vi "ConfigTriggerRequest.vi"(8 "error in (no error)":errorcluster, 10 "TriggerParams":T1={"eTrigger"=0, "eEdge"=10280, "sSource"=""} {"eEdge" items=["Rising"=10280, "Falling"=10171]; "eTrigger" items=["None", "Digital", "Analog"]}, 11 "ModuleID":i32) -> (0 "error out":errorcluster)   [LabVIEW 2014, in "FGenPlugins.lvlib" / "NISTFGenPluginsBase.lvclass"]
uses:
  NISTFGenPluginsBase.lvclass
  TypeDef/TriggerParams.ctl
  FGenModule/Protected/clEventType.ctl
  <vilib>/Utility/error.llb/Error Cluster From Error Code.vi
  <vilib>/ErrorRing/Error Ring.xnode
  FGenModule/FGenModule.lvlib
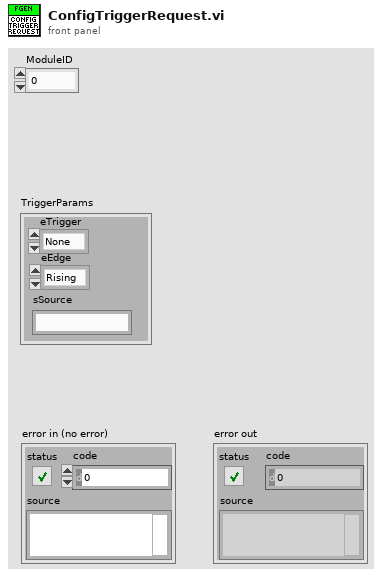
[diagram p1: front panel]
types:
  T1 = typedef "FGenPlugins.lvlib/NISTFGenPluginsBase.lvclass/TriggerParams.ctl" = cluster{"eTrigger":u16, "eEdge":u16, "sSource":string}
  T2 = typedef "FGenModule.lvlib/clRequestEvents.ctl" = cluster{"StopRequest":refnum<user-event>, "PathToINI":refnum<user-event>, " LoadPlugin":refnum<user-event>, "OperateMode":refnum<user-event>, "OutputEnable":refnum<user-event>, "OutputMode":refnum<user-event>, "RefClkSource":refnum<user-event>, "ChannelName":refnum<user-event>, "Generation":refnum<user-event>, "AbortGeneration":refnum<user-event>, "Reset":refnum<user-event>, "Initialize":refnum<user-event>, "StdWaveform":refnum<user-event>, "ClrArbWfrm":refnum<user-event>, "CreateArbWfrm":refnum<user-event>, "ConfigArbWfrm":refnum<user-event>, "ConfigArbSRat":refnum<user-event>, "GetArbWfrm":refnum<user-event>, "ConfigTriigger":refnum<user-event>, "ShowPanel":refnum<user-event>, "ReadChannelParams":refnum<user-event>, "WriteChannelParams":refnum<user-event>, "ConfigDlg":refnum<user-event>}
  T3 = typedef "FGenModule.lvlib/clEventType.ctl" = cluster{"ModuleID":i32, "Data":variant}
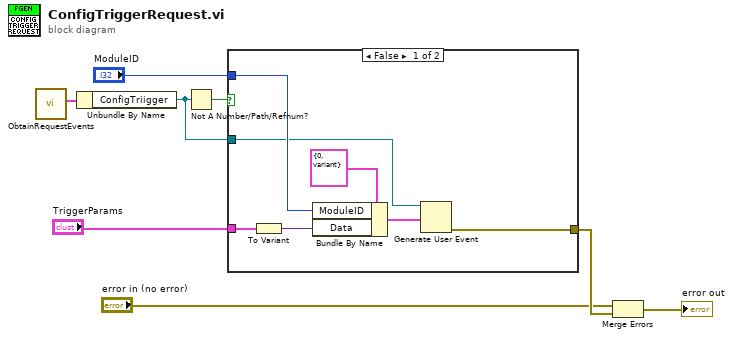
[diagram p0: block diagram]
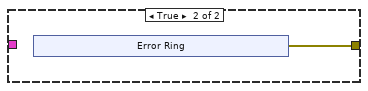
[diagram p2: hidden frame]
diagram:
  n1 = call "ObtainRequestEvents.vi"() -> ("clRequestEvents"=w8:T2)  [unwired: 10 in, 1 out]
  n2 = Unbundle By Name(w8) -> ("ConfigTriigger"=w6:refnum<user-event>)
  n3 = Not A Number/Path/Refnum?(number/path/refnum=w6) -> (NaN/Path/Refnum?=w7:bool)
  n4 = case shown="False" w7 {
    tunnel: w6 -> [w12 _]
    tunnel: "ModuleID" -> [w14 _]
    tunnel: [w11 w16] -> w3
    tunnel: "TriggerParams" -> [w9 _]
    frame False {
      n5 = To Variant(anything=w9) -> (Variant=w10:variant)
      n6 = Bundle By Name(cluster=T3 {"ModuleID"=0, "Data"=variant} ("clEventType"), "ModuleID"=w14, "Data"=w10) -> (w13:T3)
      n7 = Generate User Event(user event=w12, event data cluster=w13) -> (error out=w11:errorcluster)  [unwired: 2 in, 1 out]
    }
    frame True {
      n8 = xnode "Error Ring"() -> ("error out"=w16:errorcluster)
    }
  }
  n9 = Merge Errors("error in (no error)", w3) -> (→"error out":errorcluster)
